vi "Interpolate Ball System.vi"(8 "Duration":dbl, 9 "Current Time":dbl, 10 "End Ball System Actions":T1, 11 "Start Ball System Actions":T1) -> (3 "Ball System Actions":T1)   [LabVIEW 2019]
uses:
  Controls/Ball System Actions.ctl
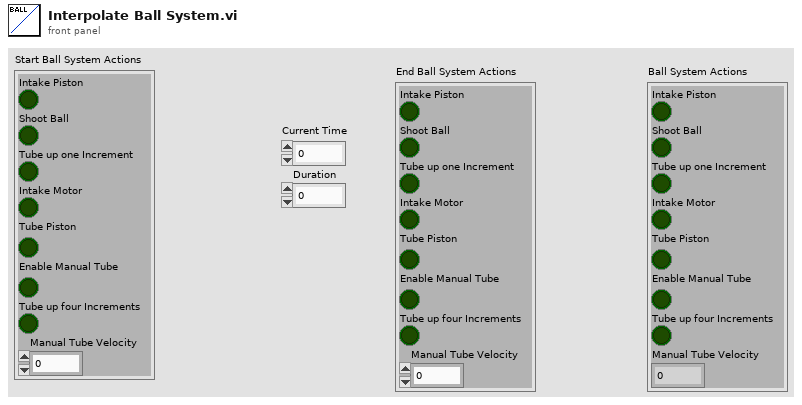
[diagram p1: front panel]
types:
  T1 = typedef "Ball System Actions.ctl" = cluster{"Intake Piston ":bool, "Shoot Ball":bool, "Tube up one Increment\t":bool, "Intake Motor\t":bool, "Tube Piston":bool, "Enable Manual Tube":bool, "Tube up four Increments":bool, "Manual Tube Velocity":dbl}
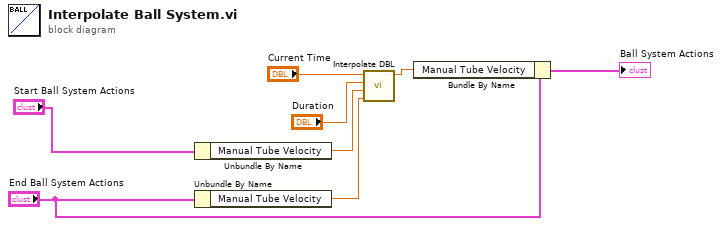
[diagram p0: block diagram]
diagram:
  n1 = Unbundle By Name("Start Ball System Actions") -> ("Manual Tube Velocity"=w6:dbl)
  n2 = Unbundle By Name("End Ball System Actions") -> ("Manual Tube Velocity"=w5:dbl)
  n3 = call "Interpolate DBL.vi"("Ending Value"=w5, "Starting Value"=w6, "Duration"="Duration", "Current Time"="Current Time") -> ("Current Value"=w4:dbl)  [unwired: 7 in]
  n4 = Bundle By Name(cluster="End Ball System Actions", "Manual Tube Velocity"=w4) -> (→"Ball System Actions":T1)
